vi "CTCGlbs.vi"() -> ()   [LabVIEW 2011]
panel:
  in  "Ext Ramp Reg":u16=201
  in  "CTC Node2":i16=1
  in  "retry":bool[](array[boolean])
  in  "timeout":bool
  in  "R Output":i32
  in  "R100":i32
  in  "Spin":i32
  in  "R107":i32
  in  "R101":i32
  in  "Filters":u16=18501
  in  "Flag Number":u16=10
  in  "Digital Reg1":u16=1001
  in  "Digital In Reg":u16=11001
  in  "Analog In Reg":u16=8500
  in  "Analog Out Reg":u16=8001
  in  "Digital Reg":u16=10001
  out "Digital States":u32
  in  "CommNum":i16=999
  in  "CTC Node":i16=1
  in  "CommType":u16(ring)=1 items=["Serial", "Network"]
  # "CTC Communication"
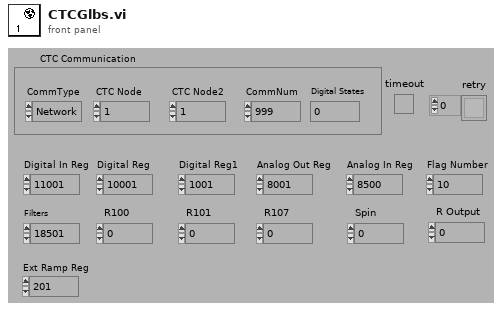
[diagram p1: front panel]
diagram:
